vi "OFDM-SIM脉冲成型.vi"(2 "error in (no error)":errorcluster, 3 "输入":cdb[](array[numeric]) caption="input", 4 "?":T1={"过采样因子"=20.0, "脉冲成形参数"={"调制类型"=enum."PSK", "脉冲成形滤波器"=enum."Raised Cosine", "滤波器参数"=0.5, "滤波长度 (码元)"=8.0}, "载波数"=128, "总比特数"=25600, "循环次数"=100, "信噪比门限/dB"=50, "M-QAM (16)"=4} {"脉冲成形参数"."滤波器参数" format="%.2f"}) -> (0 "error out":errorcluster, 1 "输出":cdb[](array[numeric]) caption="output")   [LabVIEW 2018]
uses:
  <vilib>/Analysis/2dsp.llb/1D Convolution (CDB).vi
  <vilib>/addons/Modulation/Analog/support/mod_Set Error Source.vi
  <vilib>/Analysis/2dsp.llb/Upsample (CDB).vi
  <vilib>/addons/Modulation/Digital/Support/Common/Validators/mod_Generate Filter Coefficients Validate.vi
  <vilib>/addons/Modulation/Digital/General/subVIs/mod_Generate Filter Coefficients.vi
  <vilib>/addons/Modulation/niDMT.lvlib
  <vilib>/Analysis/NI_AALPro.lvlib
panel:
  out "samples/symbol":i32
  out "pulse shaping filter coefficients":dbl[](array[numeric]) format="%.2f"
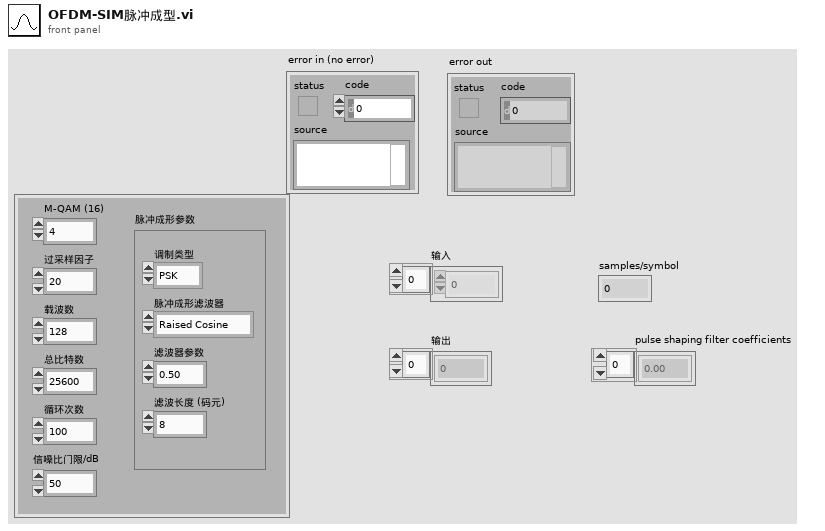
[diagram p1: front panel]
types:
  T1 = cluster{"过采样因子":dbl, "脉冲成形参数":cluster{"调制类型":enum16{"FSK", "PSK", "QAM", "MSK", "PAM", "ASK", "CPM"}, "脉冲成形滤波器":enum16{"none", "Raised Cosine", "Root Raised Cos", "Gaussian"}, "滤波器参数":dbl, "滤波长度 (码元)":dbl}, "载波数":i32, "总比特数":i32, "循环次数":i32, "信噪比门限/dB":i32, "M-QAM (16)":i32}
  T2 = cluster{"调制类型":enum16{"FSK", "PSK", "QAM", "MSK", "PAM", "ASK", "CPM"}, "脉冲成形滤波器":enum16{"none", "Raised Cosine", "Root Raised Cos", "Gaussian"}, "滤波器参数":dbl, "滤波长度 (码元)":dbl}
  T3 = enum16{"FSK", "PSK", "QAM", "MSK", "PAM", "ASK", "CPM"}
  T4 = enum16{"none", "Raised Cosine", "Root Raised Cos", "Gaussian"}
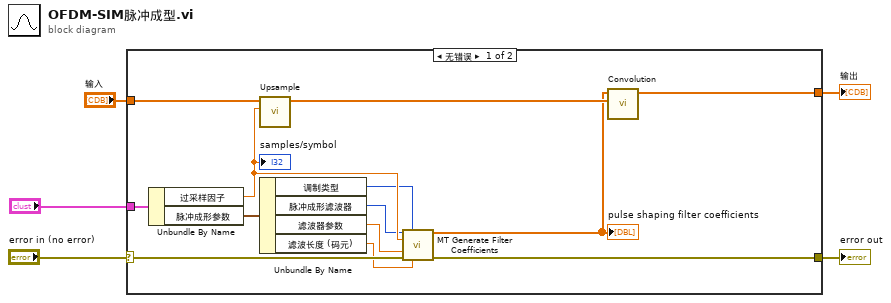
[diagram p0: block diagram]
diagram:
  n1 = case shown="无错误" "error in (no error)" {
    selector: "error in (no error)" -> [w16 w19]
    tunnel: "?" -> [w18 _]
    tunnel: [w12 w19] -> w4
    tunnel: [w7 _] -> w3
    tunnel: "输入" -> [w6 _]
    frame No Error {
      n2 = Unbundle By Name(w18) -> ("过采样因子"=w15:dbl, "脉冲成形参数"=w17:T2)
      "samples/symbol" <- w15
      n3 = call-poly <vilib>:"Upsample.vi"("upsampling factor"=w15, "X"=w6) -> ("Upsampled Array"=w14:cdb[])  [unwired: 8 in, 1 out]
      n4 = Unbundle By Name(w17) -> ("调制类型"=w11:T3, "脉冲成形滤波器"=w10:T4, "滤波器参数"=w8:dbl, "滤波长度 (码元)"=w9:dbl)
      n5 = call <vilib>:"MT Generate Filter Coefficients.vi"("pulse shaping filter (none)"=w10, "modulation type"=w11, "pulse shaping samples per symbol (16)"=w15, "filter parameter"=w8, "error in (no error)"=w16, "filter length (symbols)"=w9) -> ("pulse shaping filter coefficients"=w13:dbl[], "error out"=w12:errorcluster)  [unwired: 7 in, 1 out]
      "pulse shaping filter coefficients" <- w13
      n6 = call-poly <vilib>:"Convolution.vi"("Y"=w14, "X"=w13) -> ("X * Y"=w7:cdb[])  [unwired: 8 in, 1 out]
    }
    frame Error {
    }
  }
  "error out" <- w4
  "输出" <- w3
